vi "Don't Break the Rollers.vi"(10 "Rollers close in":bool) -> (2 "Roller close out":bool, 4 "Keeep rollers open?":bool)   [LabVIEW 2014]
uses:
  Common Code/Elevator Mode.ctl
  Common Code/Elevator State.ctl
  Robot Global Data.vi
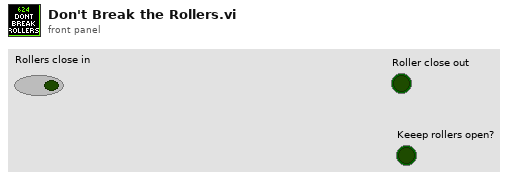
[diagram p1: front panel]
types:
  T1 = typedef "Elevator State.ctl" = enum16{"Idle", "Goto Load Position", "Wait for Load", "Load Drop", "Load Lift", "Drop Stack", "Goto Eject Position", "Eject ", "Raise Trashcan"}
  T2 = typedef "Elevator Mode.ctl" = enum16{"Manual", "Safe", "Auto"}
  T3 = typedef "Dashboard Control Data.ctl" = cluster{"Cam Exposure":dbl, "Go to angle":dbl, "Steer PID Gains":cluster{"proportional gain (Kc)":dbl, "integral time (Ti, min)":dbl, "derivative time (Td, min)":dbl}, "Steer PID output Range":cluster{"output high":dbl, "output low":dbl}, "Pressure m \nValue":dbl, "Pressure b \nValue":dbl, "Strafe Timer\nWait":dbl, "Roller Command Cluster ":T4, "Elevator":T5, "Strafe Correct max steer":dbl, "IMU Enable":bool, "Encoder Control":T7, "IMU Controls":cluster{"Pitch Zero":dbl, "Roll Zero":dbl}}
  T4 = typedef "Roller Control.ctl" = cluster{"Intake Speed":dbl, "Turn In Speed":dbl, "Unload Speed":dbl, "Turn Out Speed":dbl, "Ping Align Tolerance":dbl, "Tote Range Threshold":dbl, "Right Pot 0":dbl, "Pot Threshold":dbl, "Left Pot 0":dbl, "Manual 0s?":bool, "Right Pot Scale":dbl, "Left Pot Scale":dbl, "0 wait time":i32, "Zero Pots":bool, "Min Elevator Height":dbl, "Eject Time":dbl, "Eject US Threshold":dbl}
  T5 = typedef "Elevator DB Control.ctl" = cluster{"PID Output Range":cluster{"output high":dbl, "output low":dbl}, "PID gains":cluster{"proportional gain (Kc)":dbl, "integral time (Ti, min)":dbl, "derivative time (Td, min)":dbl}, "Height Tolerance":sgl, " Encoder Constant":dbl, "Safe Mode Max Speed":sgl, "Eject Time":sgl, "Zeroing Speed":sgl, "Presets":T6, "Ping Detect Threshold":sgl, "Use Ping?":bool}
  T6 = typedef "Elevator Presets.ctl" = cluster{"Hold Tote":sgl, "Hold Trashcan":sgl, "Pickup 2 w/ Tote":sgl, "Pickup 2 w/ Trashcan":sgl, "Pickup 3 w/ Tote":sgl, "Pickup 3 w/ Trashcan":sgl, "Bottom":sgl, "Pickup 1 w/ Tote":sgl, "Pickup Trashcan":sgl, "Pickup 1 w/ Trashcan":sgl, "Eject":sgl, "Hold 6":sgl, "Step add height":sgl, "Store Trashcan 3":sgl, "Store Trashcan 4":sgl, "Store Trashcan 5":sgl}
  T7 = typedef "Encoder Control.ctl" = cluster{"Left Tick Constant":dbl, "Right Tick Constant":dbl, "Center Tick Constant":dbl, "Reset?":bool, "Y Dist":cluster{"PID gains":cluster{"proportional gain (Kc)":dbl, "integral time (Ti, min)":dbl, "derivative time (Td, min)":dbl}, "output range":cluster{"output high":dbl, "output low":dbl}}, "X Dist":cluster{"PID gains":cluster{"proportional gain (Kc)":dbl, "integral time (Ti, min)":dbl, "derivative time (Td, min)":dbl}, "output range":cluster{"output high":dbl, "output low":dbl}}, "Y Stop Thresh":dbl, "Y Stop Speed":dbl, "X Stop Thresh":dbl, "X Stop Speed":dbl}
  T8 = typedef "Elevator Status.ctl" = cluster{"State":T1, "Eject Piston":bool, "Height":dbl, "Top Limit Switch":bool, "Bottom Limit Switch":bool, "Target":dbl, "In Range":bool, "Enc Value":dbl, "Limit Override":bool, "Mode":T2, "Stabilizer":bool, "Finger":bool, "High IR":bool, "Motor Out":dbl, "Ping Detect":bool, "Storing Trashcan?":bool}
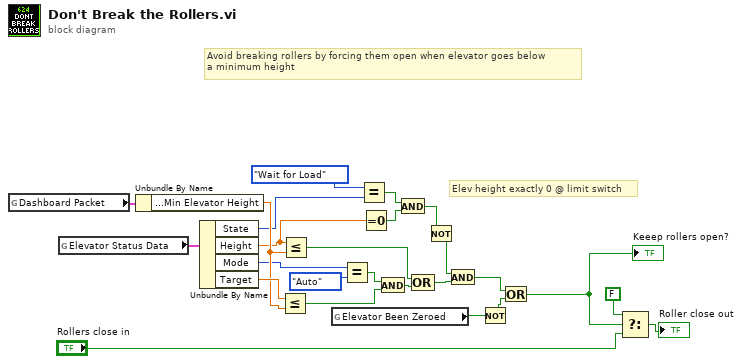
[diagram p0: block diagram]
diagram:
  # "Elev height exactly 0 @ limit switch"
  # "Avoid breaking rollers by forcing them open when elevator goes below\na minimum height"
  n1 = global read "Robot Global Data.vi" "Dashboard Packet"() -> (w24:T3)
  n2 = global read "Robot Global Data.vi" "Elevator Status Data"() -> (w25:T8)
  n3 = Unbundle By Name(w24) -> ("Roller Command Cluster.Min Elevator Height"=w22:dbl)
  n4 = Unbundle By Name(w25) -> ("State"=w6:T1, "Height"=w11:dbl, "Mode"=w21:T2, "Target"=w23:dbl)
  n5 = Less Or Equal?(x=w23, y=w22) -> (x <= y?=w18:bool)
  n6 = Less Or Equal?(x=w11, y=w22) -> (x <= y?=w16:bool)
  n7 = global read "Robot Global Data.vi" "Elevator Been Zeroed"() -> (w7:bool)
  n8 = Equal?(x=w21, y=Elevator_Mode."Auto") -> (x = y?=w19:bool)
  n9 = Equal?(x=Elevator_State."Wait for Load", y=w6) -> (x = y?=w4:bool)
  n10 = Equal To 0?(x=w11) -> (x = 0?=w3:bool)
  n11 = And(x=w19, y=w18) -> (x .and. y?=w17:bool)
  n12 = And(x=w4, y=w3) -> (x .and. y?=w2:bool)
  n13 = Compound Arithmetic op=OR(w16, w17) -> (w12:bool)
  n14 = Not(x=w2) -> (.not. x?=w1:bool)
  n15 = And(x=w1, y=w12) -> (x .and. y?=w10:bool)
  n16 = Not(x=w7) -> (.not. x?=w8:bool)
  n17 = Or(x=w10, y=w8) -> (x .or. y?=w9:bool)
  "Keeep rollers open?" <- w9
  n18 = Select(t=FALSE, s=w9, f="Rollers close in") -> (s? t:f=→"Roller close out":bool)
